vi "Load All Subitems.vi"(8 "error in (no error)":errorcluster, 11 "Application Data in":T1) -> (0 "error out":errorcluster, 3 "Application Data out":T1)   [LabVIEW 2019, in "DSF Configuration Utility.lvlib"]
uses:
  DSF Configuration Utility.lvlib
  Main VI/Application Data.ctl
  Main VI/View Mode.ctl
  VeriStand/Data Sharing Custom Device/Source/DSF Core.lvlibp/Classes/Configuration Session/Configuration Session.lvclass
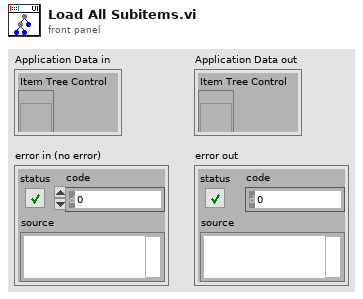
[diagram p1: front panel]
types:
  T1 = typedef "DSF Configuration Utility.lvlib/Application Data.ctl" = cluster{"Item Tree Control":refnum<vi>, "Value Tree Control":refnum<vi>, "Configuration Session":refnum<class "Configuration Session.lvclass">, "Top-Level VI":refnum<vi>, "View State":T2, "menu reference":refnum<k9>}
  T2 = typedef "DSF Configuration Utility.lvlib/View Mode.ctl" = enum16{"Tree", "List"}
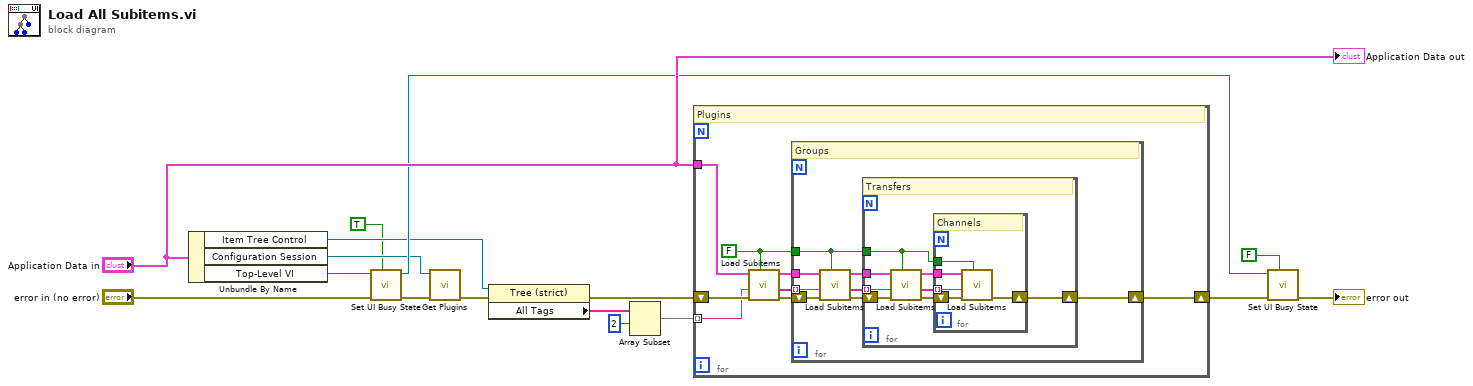
[diagram p0: block diagram]
diagram:
  n1 = Unbundle By Name("Application Data in") -> ("Item Tree Control"=w6:refnum<vi>, "Configuration Session"=w8:refnum<class "Configuration Session.lvclass">, "Top-Level VI"=w13:refnum<vi>)
  n2 = call "Set UI Busy State.vi"("Defer Panel Updates"=TRUE, "error in (no error)"="error in (no error)", "VI in"=w13) -> ("error out"=w9:errorcluster, "VI out"=w12:refnum<vi>)  [unwired: 7 in]
  n3 = call "Get Plugins.vi"("error in (no error)"=w9, "configuration session in"=w8) -> ("error out"=w7:errorcluster)  [unwired: 7 in, 2 out]
  n4 = property class="Tree (strict)"(reference=w6, error in=w7) -> (error out=w5:errorcluster, "All Tags"=w3:string[])  [unwired: 1 out]
  n5 = Array Subset(array=w3, index=2) -> (w2:string[])  [unwired: 1 in]
  n6 = for {
    tunnel: "Application Data in" -> [w24]
    tunnel: w2 -> [w17] mode=indexing
    shift-right: [w18] -> w10
    shift-left: w5 -> [w21]
    w19 = FALSE ("defer fp updates?(T)")
    # "Plugins"
    n7 = call "Load Subitems.vi"("defer fp updates?(T)"=w19, "error in (no error)"=w21, "Tag"=w17, "Application Data in"=w24) -> ("error out"=w20:errorcluster, "item children"=w23:string[], "Application Data out"=w22:T1)  [unwired: 5 in]
    n8 = for {
      tunnel: w22 -> [w32]
      tunnel: w23 -> [w31] mode=indexing
      tunnel: w19 -> [w26]
      shift-right: [w25] -> w18
      shift-left: w20 -> [w28]
      # "Groups"
      n9 = call "Load Subitems.vi"("defer fp updates?(T)"=w26, "error in (no error)"=w28, "Tag"=w31, "Application Data in"=w32) -> ("error out"=w27:errorcluster, "item children"=w29:string[], "Application Data out"=w30:T1)  [unwired: 5 in]
      n10 = for {
        tunnel: w30 -> [w40]
        tunnel: w29 -> [w37] mode=indexing
        tunnel: w26 -> [w34]
        shift-right: [w33] -> w25
        shift-left: w27 -> [w36]
        # "Transfers"
        n11 = call "Load Subitems.vi"("defer fp updates?(T)"=w34, "error in (no error)"=w36, "Tag"=w37, "Application Data in"=w40) -> ("error out"=w35:errorcluster, "item children"=w39:string[], "Application Data out"=w38:T1)  [unwired: 5 in]
        n12 = for {
          tunnel: w38 -> [w45]
          tunnel: w39 -> [w44] mode=indexing
          tunnel: w34 -> [w41]
          shift-right: [w42] -> w33
          shift-left: w35 -> [w43]
          # "Channels"
          n13 = call "Load Subitems.vi"("defer fp updates?(T)"=w41, "error in (no error)"=w43, "Tag"=w44, "Application Data in"=w45) -> ("error out"=w42:errorcluster)  [unwired: 5 in, 2 out]
        }
      }
    }
  }
  n14 = call "Set UI Busy State.vi"("Defer Panel Updates"=FALSE, "error in (no error)"=w10, "VI in"=w12) -> ("error out"=→"error out":errorcluster)  [unwired: 7 in, 1 out]
  "Application Data out" <- "Application Data in"
